vi "clear_buffers.vi"(8 "error in (no error)":errorcluster, 11 "FPGAWrapperMH120124RAPS_PXI7813R in":refnum<class "FPGAWrapperMH120124RAPS_PXI7813R.lvclass">) -> (0 "error out":errorcluster, 3 "FPGAWrapperMH120124RAPS_PXI7813R out":refnum<class "FPGAWrapperMH120124RAPS_PXI7813R.lvclass">)   [LabVIEW 2010, in "FPGAWrapperMH120124RAPS_PXI7813R.lvclass"]
uses:
  FPGAWrapperMH120124RAPS_PXI7813R.lvclass
  grabber/command_enum.ctl
  class_data.vi
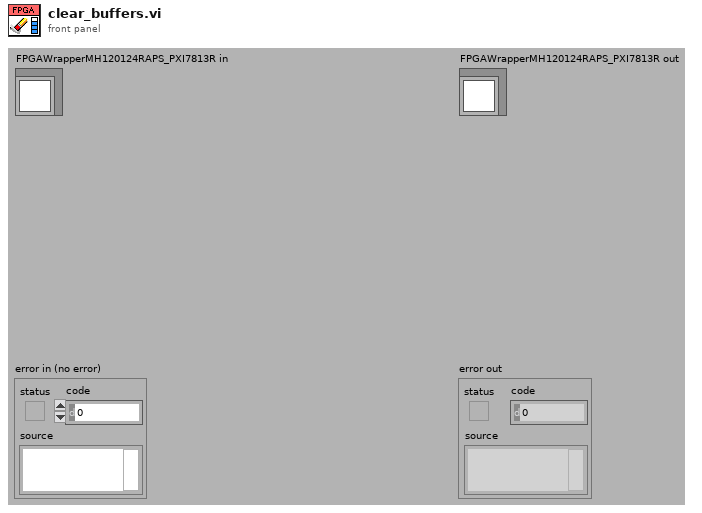
[diagram p1: front panel]
types:
  T1 = typedef "command_enum.ctl" = enum8{"NULL", "update", "start", "stop", "reset", "shut-down"}
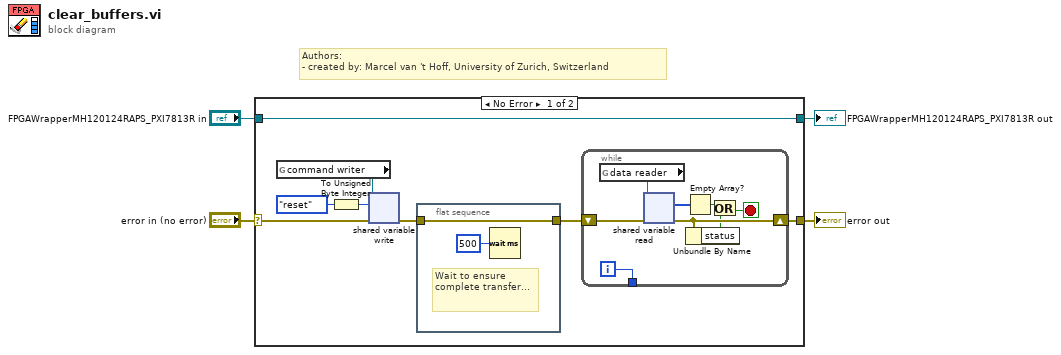
[diagram p0: block diagram]
diagram:
  # "Authors: \n- created by: Marcel van 't Hoff, University of Zurich, Switzerland"
  n1 = case shown="No Error" "error in (no error)" {
    selector: "error in (no error)" -> [w9 w23]
    tunnel: [w8 w23] -> w2
    tunnel: [w12 w24] -> w1
    tunnel: "FPGAWrapperMH120124RAPS_PXI7813R in" -> [w12 w24]
    frame No Error {
      n2 = global read "class_data.vi" "command writer"() -> (w5:refnum<k21>)
      n3 = To Unsigned Byte Integer(number=command_enum."reset" ("command")) -> (unsigned 8bit integer=w6:u8)
      n4 = shared-variable-write(w5, w9, w6) -> (w10:errorcluster)  [unwired: 1 in, 2 out]
      n5 = flat-sequence {
        tunnel: w10 -> [w22]
        tunnel: [w22] -> w11
        frame #0 {
          # "Wait to ensure complete transfer..."
          n6 = Wait (ms)(milliseconds to wait=u32 500) -> ()  [unwired: 1 out]
        }
      }
      n7 = while {
        shift-right: [w17] -> w8
        shift-left: w11 -> [w20]
        tunnel: [w13] -> _
        i -> [w13]
        stop <- w14 stop-if-true
        n8 = global read "class_data.vi" "data reader"() -> (w19:refnum<k21>)
        n9 = shared-variable-read(w19, w20) -> (w17:errorcluster, w18:u64[])  [unwired: 2 in, 2 out]
        n10 = Empty Array?(array=w18) -> (empty?=w15:bool)
        n11 = Unbundle By Name(w17) -> ("status"=w16:bool)
        n12 = Or(x=w15, y=w16) -> (x .or. y?=w14:bool)
      }
    }
    frame Error {
    }
  }
  "error out" <- w2
  "FPGAWrapperMH120124RAPS_PXI7813R out" <- w1
